vi "Visualize LiDAR data.vi"(11 "Input LiDAR":T1) -> (3 "Array":cluster{"x LiDAR":dbl[], "y LiDAR":dbl[]}[](array[cluster]))   [LabVIEW 2016]
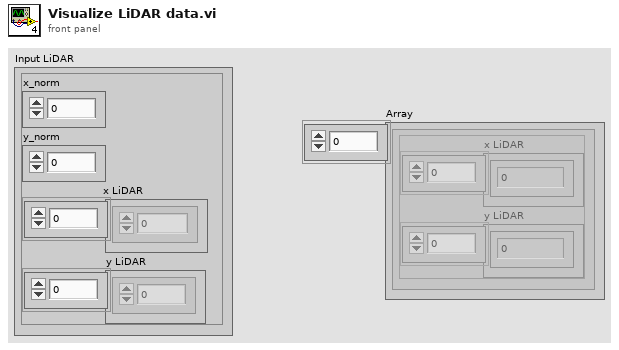
[diagram p1: front panel]
types:
  T1 = cluster{"x_norm":dbl, "y_norm":dbl, "x LiDAR":dbl[], "y LiDAR":dbl[]}
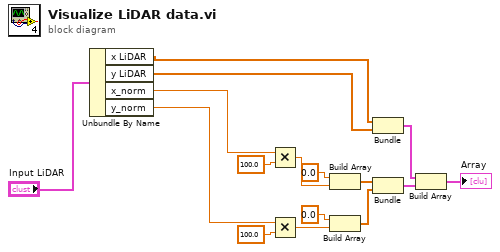
[diagram p0: block diagram]
diagram:
  n1 = Unbundle By Name("Input LiDAR") -> ("x LiDAR"=w4:dbl[], "y LiDAR"=w3:dbl[], "x_norm"=w2:dbl, "y_norm"=w1:dbl)
  n2 = Multiply(x=w2, y=100.0) -> (x*y=w8:dbl)
  n3 = Multiply(x=w1, y=100.0) -> (x*y=w11:dbl)
  n4 = Build Array(0.0 ("element"), w8) -> (w13:dbl[])
  n5 = Build Array(0.0 ("element"), w11) -> (w12:dbl[])
  n6 = Bundle("x LiDAR"=w4, "y LiDAR"=w3) -> (w14:cluster{"x LiDAR":dbl[], "y LiDAR":dbl[]})  [unwired: 1 in]
  n7 = Bundle(w13, w12) -> (w16:cluster{dbl[], dbl[]})  [unwired: 1 in]
  n8 = Build Array(w14, w16) -> (→"Array":cluster{"x LiDAR":dbl[], "y LiDAR":dbl[]}[])
